vi "Calculate Controler Vin.vi"(8 "error in (no error)":errorcluster, 10 "Acquisition Context":T1, 11 "Stimulus Settings":T2) -> (0 "error out":errorcluster, 3 "Vin":dbl)   [LabVIEW 2026, in "Acquisition.lvlib"]
uses:
  Acquisition.lvlib
  controls/Controller/Stimulus Settings.ctl
  controls/Controller/Stimulus Outputs.ctl
  controls/Controller/Stimulus Output.ctl
  controls/Controller/Controller Core Data.ctl
  controls/UI/Units Enum.ctl
  controls/UI/Signal Enum.ctl
  controls/Controller/Stimulus Output Configuration.ctl
  controls/Controller/Stimulus Role.ctl
  Acquisition Context.ctl
  Settings/Settings.lvlib
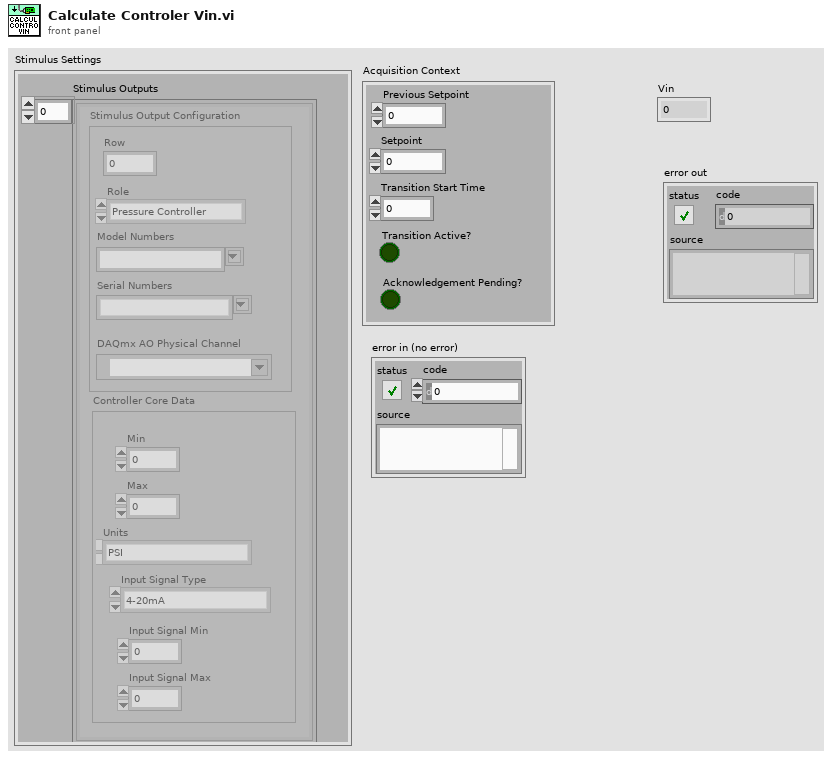
[diagram p1: front panel]
types:
  T1 = typedef "Acquisition.lvlib/Acquisition Context.ctl" = cluster{"Setpoint":dbl, "Previous Setpoint":dbl, "Transition Start Time":dbl, "Transition Active?":bool, "Acknowledgement Pending?":bool}
  T2 = typedef "Settings.lvlib/Stimulus Settings.ctl" = cluster{"Stimulus Outputs":T3}
  T3 = typedef "Settings.lvlib/Stimulus Outputs.ctl" = T4[]
  T4 = typedef "Settings.lvlib/Stimulus Output.ctl" = cluster{"Controller Core Data":T5, "Stimulus Output Configuration":T8}
  T5 = typedef "Settings.lvlib/Controller Core Data.ctl" = cluster{"Min":dbl, "Max":dbl, "Units":T6, "Input Signal Type":T7, "Input Signal Min":dbl, "Input Signal Max":dbl}
  T6 = typedef "Units Enum.ctl" = enum16{"PSI", "Deg C", "kPa", "GPM"}
  T7 = typedef "Signal Enum.ctl" = enum16{"4-20mA", "0-10V", "Thermocouple Type K"}
  T8 = typedef "Settings.lvlib/Stimulus Output Configuration.ctl" = cluster{"DAQmx AO Physical Channel":tag, "Role":T9, "Model Numbers":string, "Serial Numbers":string, "Row":i32}
  T9 = typedef "Stimulus Role.ctl" = enum16{"Pressure Controller", "Temperature Controller"}
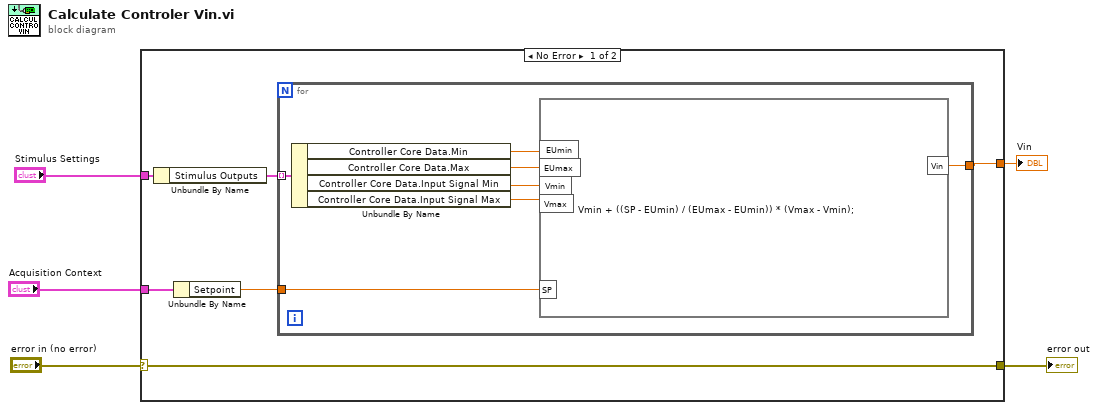
[diagram p0: block diagram]
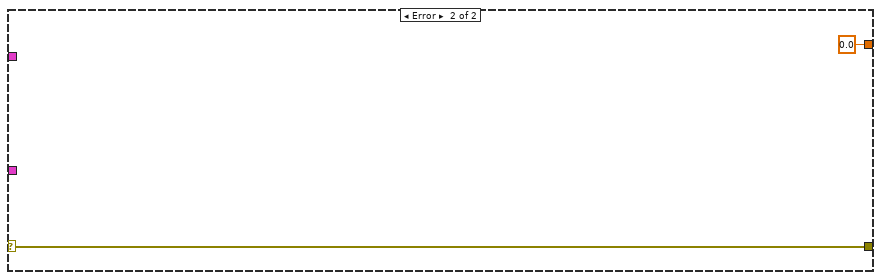
[diagram p2: hidden frame]
diagram:
  n1 = case shown="No Error" "error in (no error)" {
    selector: "error in (no error)" -> [w6 w19]
    tunnel: "Stimulus Settings" -> [w11 _]
    tunnel: "Acquisition Context" -> [w9 _]
    tunnel: [w7 0.0 ("Vin")] -> w3
    tunnel: [w6 w19] -> w1
    frame No Error {
      n2 = Unbundle By Name(w11) -> ("Stimulus Outputs"=w10:T3)
      n3 = Unbundle By Name(w9) -> ("Setpoint"=w8:dbl)
      n4 = for {
        tunnel: w10 -> [w18] mode=indexing
        tunnel: w8 -> [w17]
        tunnel: [w16] -> w7
        n5 = Unbundle By Name(w18) -> ("Controller Core Data.Min"=w13:dbl, "Controller Core Data.Max"=w12:dbl, "Controller Core Data.Input Signal Min"=w15:dbl, "Controller Core Data.Input Signal Max"=w14:dbl)
        n6 = formula code="Vin = Vmin + ((SP - EUmin) / (EUmax - EUmin)) * (Vmax - Vmin);"("Vmin"=w15, "SP"=w17, "EUmin"=w13, "EUmax"=w12, "Vmax"=w14) -> ("Vin"=w16:dbl)
      }
    }
    frame Error {
    }
  }
  "error out" <- w1
  "Vin" <- w3
